vi "Read Lidar Data.vi"(8 "error in (no error)":errorcluster) -> (0 "error out":errorcluster, 2 "Direction":dbl[](array[numeric]), 3 "Magnitude":dbl[](array[numeric]))   [LabVIEW 2017]
uses:
  Variables/Labview lidar globals.vi
  <instrlib>/Hokuyo URG Series/Hokuyo URG Series.lvlib
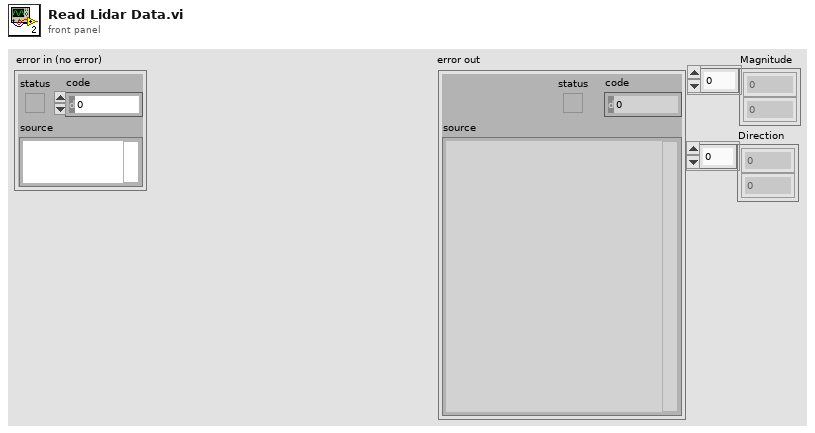
[diagram p1: front panel]
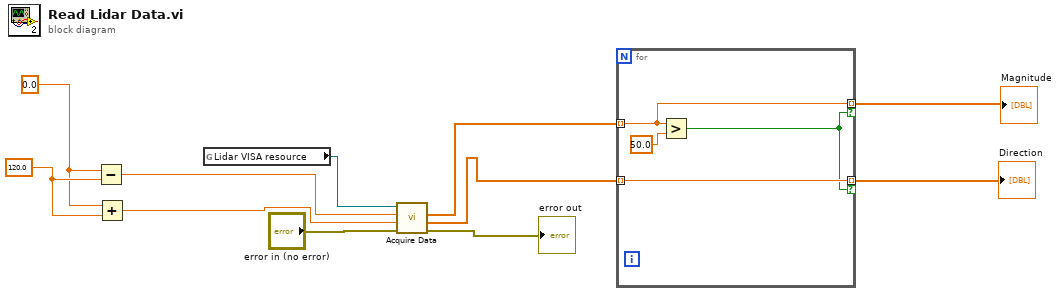
[diagram p0: block diagram]
diagram:
  w8 = 120.0 ("y")
  w7 = 0.0 ("Start Point (-120°)")
  n1 = Subtract(x=w7, y=w8) -> (x-y=w5:dbl)
  n2 = Add(x=w7, y=w8) -> (x+y=w6:dbl)
  n3 = global read "Labview lidar globals.vi" "Lidar VISA resource"() -> (w9:refnum<visa-resource-name>)
  n4 = call <instrlib>:"Acquire Data.vi"("error in (no error)"="error in (no error)", "End Point (120°)"=w6, "Start Point (-120°)"=w5, "VISA resource name"=w9) -> ("error out"=→"error out":errorcluster, "Direction"=w1:dbl[], "Magnitude"=w4:dbl[])  [unwired: 4 in, 1 out]
  n5 = for {
    tunnel: w4 -> [w14] mode=indexing
    tunnel: w1 -> [w13] mode=indexing
    tunnel: [w14] -> w3 mode=indexing if=w12
    tunnel: [w13] -> w2 mode=indexing if=w12
    n6 = Greater?(x=w14, y=50.0) -> (0:w12:bool)
  }
  "Magnitude" <- w3
  "Direction" <- w2
